vi "ConfigDlg.vi"(8 "error in (no error)":errorcluster, 11 "FitterBase in":refnum<class "FitterBase.lvclass">) -> (0 "error out":errorcluster, 2 "Changed":bool, 3 "FitterBase out":refnum<class "FitterBase.lvclass">)   [LabVIEW 2014, in "AnalysisPlugins.lvlib" / "FitterBase.lvclass"]
uses:
  FitterBase.lvclass
  AnalysisPluginBaseClass/AnalysisPluginsBase.lvclass
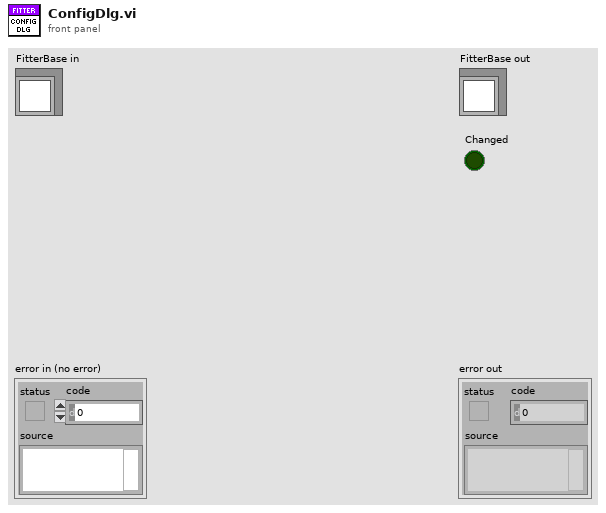
[diagram p1: front panel]
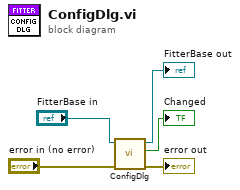
[diagram p0: block diagram]
diagram:
  n1 = call-parent "ConfigDlg.vi"("error in (no error)"="error in (no error)", "AnalysisPluginsBase in"="FitterBase in") -> ("error out"=→"error out":errorcluster, "Changed"=→"Changed":bool, "AnalysisPluginsBase out"=→"FitterBase out":refnum<class "FitterBase.lvclass">)  [unwired: 7 in]
